vi "PART_II_main.vi"() -> ()   [LabVIEW 2019]
uses:
  <vilib>/Math Plots/3D Math Plots/3D Mesh/3D Mesh XCtrl/3D Mesh.xctl
  <vilib>/Math Plots/3D Math Plots/3D Mesh/3D Mesh Datatype/3D Mesh Datatype.lvclass
  <vilib>/Math Plots/3D Math Plots/3D Mesh/3D Mesh Datatype/Public/Plot Helper (Matrix).vi
panel:
  in  "numbinsX":dbl=20.0
  in  "minX":dbl=-40.0
  in  "maxX":dbl=40.0
  out "3D Mesh":refnum<class "3D Plot Datatype.lvclass">[](xcontrol)
  out "1D Histogram X":dbl[](graph)=[0.0, 0.0, 0.0, 0.0, 0.0, 0.0, 1.0, 12.0, 25.0, 47.0, 142.0, 271.0, 270.0, 113.0, 34.0, 27.0, 12.0, 6.0, 4.0, 3.0]
  out "Waveform Graph Raw Data":dbl[][](graph)
  out "Rounded and Rescaled Data":dbl[](graph)=[12.0, 13.0, 13.0, 12.0, 12.0, 12.0, 12.0, 11.0, 11.0, 10.0, 8.0, 8.0, 8.0, 8.0, 8.0, 8.0, 9.0, 9.0, 9.0, 10.0, 11.0, 12.0, 12.0, 13.0, 13.0, 13.0, 13.0, 13.0, 13.0, 13.0, 12.0, 11.0, 11.0, 10.0, 9.0, 8.0, 8.0, 8.0, 8.0, 9.0, 9.0, 9.0, 8.0, 8.0, 9.0, 9.0, 10.0, 11.0, 11.0, 12.0, 13.0, 13.0, 13.0, 13.0, 13.0, 12.0, 12.0, 12.0, 10.0, 10.0, 9.0, 9.0, 9.0, 8.0, 9.0, 9.0, 9.0, 10.0, 11.0, 11.0, 10.0, 9.0, 8.0, 8.0, 8.0, 7.0, 8.0, 9.0, 11.0, 12.0, 12.0, 14.0, 15.0, 15.0, 15.0, 15.0, 14.0, 13.0, 12.0, 10.0, 9.0, 8.0, 7.0, 7.0, 6.0, 6.0, 6.0, 6.0, 8.0, 9.0, 10.0, 11.0, 12.0, 13.0, 14.0, 14.0, 15.0, 14.0, 13.0, 12.0, 12.0, 11.0, 10.0, 10.0, 9.0, 8.0, 8.0, 8.0, 7.0, 6.0, 6.0, 7.0, 7.0, 9.0, 9.0, 11.0, 12.0, 12.0, 12.0, 14.0, 14.0, 14.0, 13.0, 13.0, 12.0, 11.0, 10.0, 9.0, 7.0, 7.0, 7.0, 7.0, 6.0, 6.0, 7.0, 7.0, 8.0, 9.0, 10.0, 12.0, 13.0, 12.0, 13.0, 14.0, 13.0, 12.0, 12.0, 11.0, 10.0, 10.0, 9.0, 9.0, 9.0, 7.0, 7.0, 7.0, 7.0, 8.0, 8.0, 10.0, 10.0, 11.0, 12.0, 14.0, 15.0, 15.0, 14.0, 14.0, 13.0, 12.0, 10.0, 10.0, 9.0, 7.0, 6.0, 7.0, 7.0, 7.0, 7.0, 8.0, 9.0, 10.0, 11.0, 11.0, 13.0, 14.0, 15.0, 15.0, 14.0, 14.0, 12.0, 12.0, 12.0, 11.0, 9.0, 9.0, 7.0, 6.0, 6.0, 6.0, 6.0, 7.0, 8.0, 8.0, 9.0, 10.0, 11.0, 13.0, 13.0, 13.0, 13.0, 14.0, 14.0, 15.0, 15.0, 14.0, 12.0, 12.0, 10.0, 8.0, 7.0, 7.0, 5.0, 7.0, 8.0, 8.0, 9.0, 10.0, 11.0, 11.0, 12.0, 11.0, 10.0, 11.0, 10.0, 9.0, 11.0, 11.0, 9.0, 9.0, 10.0, 10.0, 10.0, 10.0, 9.0, 9.0, 9.0, 12.0, 12.0, 11.0, 10.0, 10.0, 10.0, 9.0, 12.0, 9.0, 9.0, 9.0, 10.0, 9.0, 9.0, 8.0, 9.0, 9.0, 10.0, 11.0, 12.0, 12.0, 12.0, 11.0, 12.0, 12.0, 12.0, 11.0, 10.0, 8.0, 8.0, 8.0, 8.0, 8.0, 8.0, 10.0, 10.0, 12.0, 12.0, 13.0, 13.0, 13.0, 13.0, 11.0, 11.0, 12.0, 9.0, 8.0, 8.0, 9.0, 7.0, 6.0, 8.0, 8.0, 10.0, 12.0, 12.0, 14.0, 14.0, 13.0, 11.0, 12.0, 12.0, 10.0, 10.0, 11.0, 8.0, 9.0, 8.0, 8.0, 8.0, 8.0, 8.0, 8.0, 11.0, 12.0, 13.0, 12.0, 11.0, 12.0, 12.0, 12.0, 13.0, 13.0, 11.0, 9.0, 7.0, 8.0, 7.0, 6.0, 6.0, 7.0, 8.0, 8.0, 11.0, 12.0, 13.0, 14.0, 13.0, 13.0, 13.0, 12.0, 11.0, 11.0, 10.0, 10.0, 10.0, 9.0, 7.0, 8.0, 8.0, 8.0, 8.0, 8.0, 9.0, 10.0, 11.0, 12.0, 11.0, 10.0, 11.0, 11.0, 11.0, 12.0, 10.0, 8.0, 8.0, 8.0, 7.0, 7.0, 7.0, 8.0, 10.0, 12.0, 14.0, 13.0, 14.0, 13.0, 12.0, 10.0, 11.0, 10.0, 8.0, 7.0, 7.0, 7.0, 7.0, 7.0, 8.0, 9.0, 11.0, 12.0, 13.0, 11.0, 12.0, 13.0, 11.0, 10.0, 11.0, 11.0, 10.0, 8.0, 9.0, 8.0, 7.0, 7.0, 7.0, 7.0, 8.0, 9.0, 11.0, 12.0, 12.0, 13.0, 11.0, 11.0, 12.0, 12.0, 11.0, 12.0, 11.0, 9.0, 7.0, 7.0, 7.0, 7.0, 8.0, 8.0, 8.0, 9.0, 11.0, 12.0, 12.0, 12.0, 12.0, 11.0, 12.0, 12.0, 12.0, 13.0, 12.0, 11.0, 9.0, 8.0, 6.0, 6.0, 6.0, 6.0, 7.0, 7.0, 10.0, 11.0, 12.0, 13.0, 13.0, 12.0, 13.0, 12.0, 12.0, 11.0, 10.0, 9.0, 8.0, 7.0, 8.0, 8.0, 8.0, 9.0, 9.0, 9.0, 10.0, 12.0, 12.0, 11.0, 11.0, 12.0, 12.0, 11.0, 12.0, 11.0, 9.0, 7.0, 7.0, 7.0, 6.0, 6.0, 7.0, 8.0, 9.0, 11.0, 13.0, 12.0, 12.0, 12.0, 12.0, 11.0, 11.0, 11.0, 10.0, 11.0, 11.0, 8.0, 8.0, 8.0, 8.0, 7.0, 7.0, 8.0, 8.0, 10.0, 11.0, 10.0, 12.0, 12.0, 11.0, 11.0, 12.0, 12.0, 11.0, 11.0, 11.0, 9.0, 8.0, 8.0, 7.0, 6.0, 6.0, 8.0, 8.0, 8.0, 10.0, 10.0, 13.0, 13.0, 13.0, 13.0, 13.0, 12.0, 11.0, 10.0, 9.0, 8.0, 7.0, 8.0, 7.0, 7.0, 7.0, 8.0, 9.0, 9.0, 11.0, 11.0, 12.0, 13.0, 13.0, 13.0, 12.0, 12.0, 11.0, 11.0, 10.0, 8.0, 8.0, 6.0, 6.0, 6.0, 7.0, 7.0, 9.0, 10.0, 11.0, 11.0, 13.0, 13.0, 13.0, 13.0, 12.0, 12.0, 11.0, 11.0, 10.0, 8.0, 7.0, 7.0, 7.0, 6.0, 8.0, 8.0, 8.0, 10.0, 10.0, 10.0, 11.0, 12.0, 12.0, 12.0, 12.0, 12.0, 12.0, 12.0, 11.0, 10.0, 9.0, 6.0, 6.0, 5.0, 6.0, 6.0, 7.0, 9.0, 9.0, 11.0, 13.0, 13.0, 13.0, 13.0, 12.0, 12.0, 12.0, 12.0, 11.0, 10.0, 9.0, 7.0, 3.0, 8.0, 7.0, 7.0, 7.0, 7.0, 8.0, 9.0, 10.0, 10.0, 11.0, 12.0, 12.0, 12.0, 13.0, 14.0, 12.0, 11.0, 10.0, 9.0, 7.0, 6.0, 5.0, 5.0, 6.0, 7.0, 8.0, 9.0, 11.0, 11.0, 11.0, 13.0, 13.0, 13.0, 12.0, 12.0, 12.0, 12.0, 12.0, 12.0, 10.0, 9.0, 8.0, 8.0, 5.0, 6.0, 6.0, 6.0, 7.0, 8.0, 8.0, 10.0, 11.0, 12.0, 13.0, 13.0, 14.0, 13.0, 13.0, 12.0, 12.0, 11.0, 9.0, 9.0, 8.0, 9.0, 6.0, 8.0, 7.0, 8.0, 8.0, 8.0, 9.0, 10.0, 12.0, 13.0, 13.0, 12.0, 13.0, 14.0, 14.0, 13.0, 12.0, 10.0, 9.0, 8.0, 8.0, 6.0, 6.0, 5.0, 6.0, 7.0, 8.0, 10.0, 11.0, 12.0, 13.0, 13.0, 13.0, 13.0, 12.0, 12.0, 11.0, 11.0, 10.0, 9.0, 8.0, 7.0, 6.0, 6.0, 6.0, 7.0, 6.0, 7.0, 9.0, 9.0, 10.0, 11.0, 12.0, 14.0, 14.0, 14.0, 12.0, 12.0, 11.0, 10.0, 8.0, 7.0, 7.0, 5.0, 5.0, 6.0, 7.0, 8.0, 8.0, 9.0, 11.0, 13.0, 13.0, 13.0, 13.0, 13.0, 13.0, 12.0, 12.0, 10.0, 9.0, 7.0, 6.0, 6.0, 5.0, 5.0, 6.0, 8.0, 8.0, 10.0, 11.0, 12.0, 12.0, 13.0, 12.0, 12.0, 12.0, 11.0, 11.0, 11.0, 11.0, 12.0, 9.0, 8.0, 8.0, 7.0, 5.0, 7.0, 7.0, 7.0, 9.0, 9.0, 11.0, 12.0, 13.0, 13.0, 13.0, 13.0, 13.0, 13.0, 12.0, 10.0, 9.0, 9.0, 8.0, 8.0, 6.0, 6.0, 7.0, 7.0, 8.0, 9.0, 11.0, 12.0, 12.0, 13.0, 12.0, 13.0, 13.0, 13.0, 12.0, 11.0, 11.0, 10.0, 8.0, 8.0, 7.0, 6.0, 6.0, 7.0, 7.0, 8.0, 9.0, 10.0, 11.0, 11.0, 12.0, 12.0, 12.0, 12.0, 12.0, 12.0, 12.0, 12.0, 11.0, 10.0, 10.0, 8.0, 8.0, 7.0, 6.0, 7.0, 7.0, 7.0, 8.0, 8.0, 9.0, 10.0, 10.0, 12.0, 12.0, 12.0, 12.0, 12.0, 12.0, 12.0, 12.0, 11.0, 9.0, 9.0, 8.0, 7.0, 6.0, 6.0, 7.0, 7.0, 10.0, 11.0, 11.0, 11.0, 11.0, 11.0, 11.0, 10.0, 10.0, 11.0, 11.0, 10.0, 9.0, 9.0, 9.0, 9.0, 9.0, 9.0, 8.0, 8.0, 10.0, 10.0, 11.0, 12.0, 12.0, 13.0, 12.0, 12.0, 12.0, 12.0, 11.0, 10.0, 8.0, 6.0, 6.0, 5.0, 5.0, 7.0, 8.0, 9.0, 12.0, 12.0, 13.0, 13.0, 13.0, 13.0, 11.0, 10.0, 9.0, 8.0, 8.0, 8.0, 9.0, 10.0, 10.0, 10.0, 10.0, 10.0, 10.0, 10.0, 10.0, 10.0, 10.0, 10.0, 10.0]
  in  "numbinsY":dbl=20.0
  in  "minY":dbl=-40.0
  in  "maxY":dbl=40.0
  in  "Acceleration Raw Data":dbl[][](array[numeric])=array967x6[5802 elements]
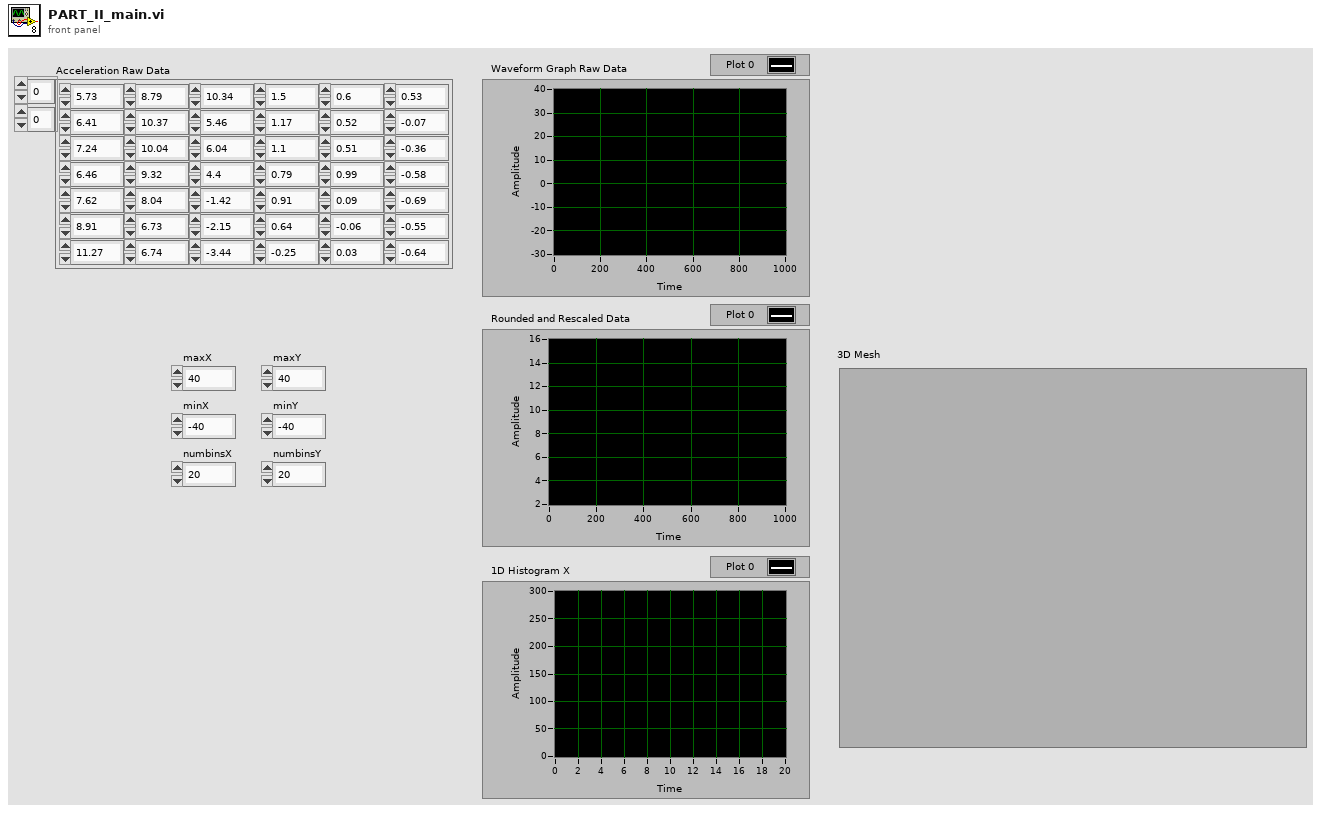
[diagram p1: front panel]
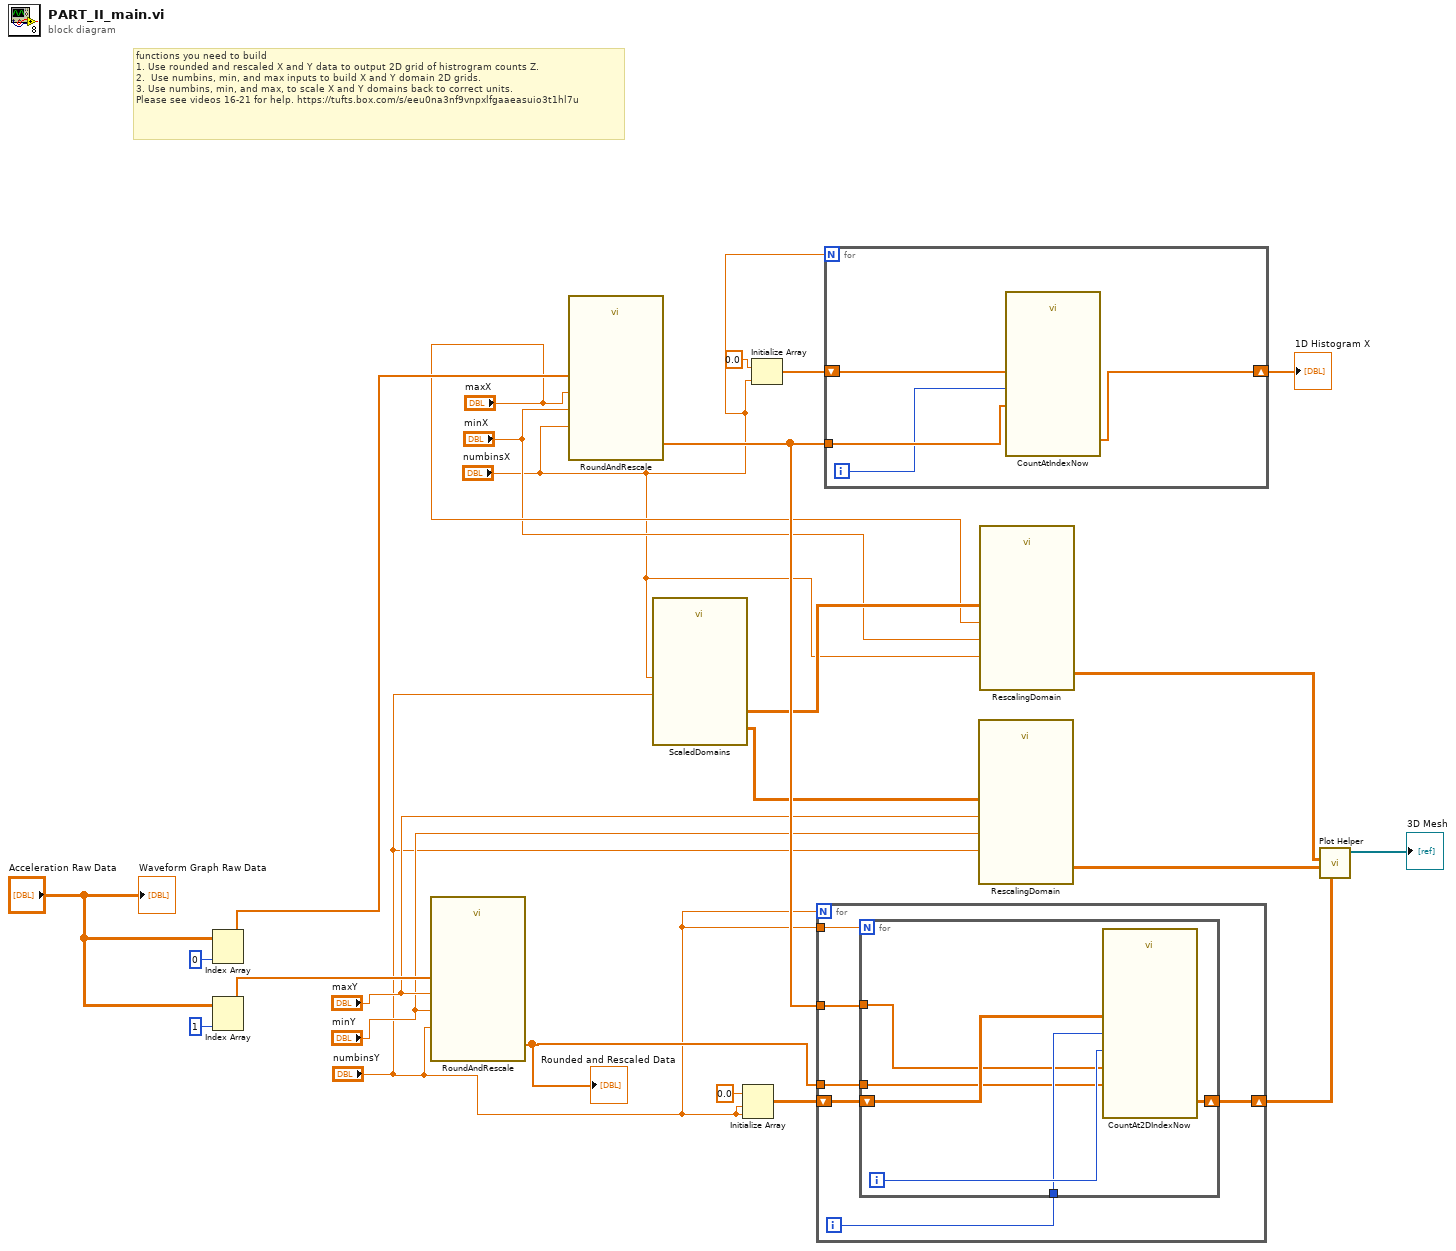
[diagram p0: block diagram]
diagram:
  # "functions you need to build\n1. Use rounded and rescaled X and Y data to output 2D grid of histrogram counts Z.\n2.  Use numbins, min, and max inputs to build X and Y domain 2D grids.\n3. Use numbins, min, and max, to scale X and Y domains back to correct units.\nPlease see videos 16-21 for help. https://tufts.box.com/s/eeu0na3nf9vnpxlfgaaeasuio3t1hl7u"
  n1 = Index Array "Index Array"(array="Acceleration Raw Data", index (col)=0 ("disabled index (col)")) -> (element=w15:dbl[])  [unwired: 1 in]
  n2 = Index Array "Index Array"(array="Acceleration Raw Data", index (col)=1 ("disabled index (col)")) -> (element=w20:dbl[])  [unwired: 1 in]
  n3 = call "RoundAndRescale.vi"("maxX"="maxY", "minX"="minY", "all rows"=w20, "numbins"="numbinsY") -> ("RoundedArray"=w16:dbl[])  [unwired: 7 in]
  "Rounded and Rescaled Data" <- w16
  n4 = call "RoundAndRescale.vi"("maxX"="maxX", "minX"="minX", "all rows"=w15, "numbins"="numbinsX") -> ("RoundedArray"=w11:dbl[])  [unwired: 7 in]
  n5 = call "ScaledDomains.vi"("numbinsY"="numbinsY", "numbinsX"="numbinsX") -> ("YDomainScaled"=w8:dbl[][], "XDomainScaled"=w7:dbl[][])  [unwired: 8 in]
  n6 = Initialize Array(0.0 ("element"), "numbinsY", "numbinsY") -> (w18:dbl[][])
  n7 = Initialize Array(0.0 ("element"), "numbinsX") -> (w13:dbl[])
  n8 = for {
    N: "numbinsY" -> [_]
    shift-right: [w30] -> w19
    shift-left: w18 -> [w29]
    tunnel: "numbinsY" -> [w27]
    tunnel: w16 -> [w26]
    tunnel: w11 -> [w25]
    i -> [w28]
    n9 = for {
      N: w27 -> [_]
      shift-right: [w36] -> w30
      shift-left: w29 -> [w35]
      tunnel: w28 -> [w33]
      tunnel: w26 -> [w32]
      tunnel: w25 -> [w31]
      i -> [w34]
      n10 = call "CountAt2DIndexNow.vi"("Rounded Y Array"=w32, "Index Y"=w34, "Rounded X Array"=w31, "Index X"=w33, "Bin 2D array in"=w35) -> ("Bin 2D array out"=w36:dbl[][])  [unwired: 6 in]
    }
  }
  n11 = for {
    N: "numbinsX" -> [_]
    tunnel: w11 -> [w40]
    shift-right: [w37] -> w12
    shift-left: w13 -> [w38]
    i -> [w39]
    n12 = call "CountAtIndexNow.vi"("Index Now"=w39, "RoundedArray"=w40, "hist box in"=w38) -> ("hist box out"=w37:dbl[])  [unwired: 7 in, 1 out]
  }
  "1D Histogram X" <- w12
  n13 = call "RescalingDomain.vi"("min"="minY", "max"="maxY", "numbins"="numbinsY", "Domain"=w8) -> ("RescaledDomain"=w10:dbl[][])  [unwired: 7 in]
  n14 = call "RescalingDomain.vi"("min"="minX", "max"="maxX", "numbins"="numbinsX", "Domain"=w7) -> ("RescaledDomain"=w9:dbl[][])  [unwired: 7 in]
  n15 = call-poly <vilib>:"Plot Helper.vi"("z matrix"=w19, "y matrix"=w10, "x matrix"=w9) -> ("3D Plot lvclass Array out"=→"3D Mesh":refnum<class "3D Plot Datatype.lvclass">[])  [unwired: 3 in, 5 out]
  "Waveform Graph Raw Data" <- "Acceleration Raw Data"
